vi "FPGA Triggered.vi"(8 "Action":T1, 11 "Input":bool) -> (2 "FPGA Triggered?":bool)   [LabVIEW 2013]
uses:
  <userlib>/Accelerator/Global Variables/Action Items.ctl
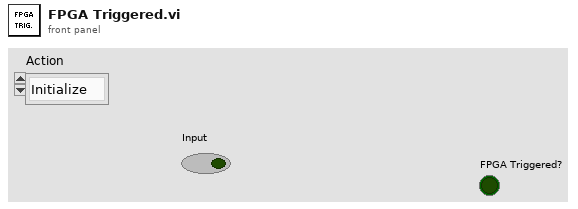
[diagram p1: front panel]
types:
  T1 = typedef "Action Items.ctl" = enum16{"Initialize", "Get", "Set"}
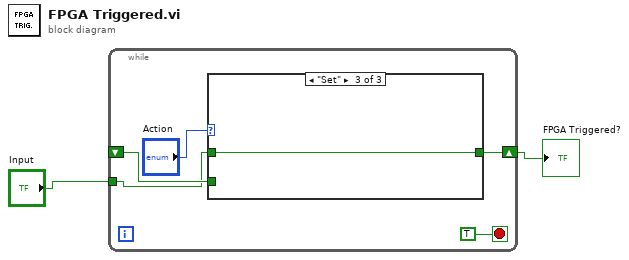
[diagram p0: block diagram]
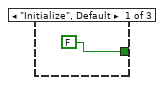
[diagram p2: hidden frame]
diagram:
  n1 = while {
    shift-right: [w5] -> w2
    shift-left: _ -> [w4]
    tunnel: "Input" -> [w3]
    stop <- TRUE stop-if-true
    n2 = case shown="\"Set\"" "Action" {
      tunnel: [FALSE w9 w10] -> w5
      tunnel: w4 -> [_ w9 _]
      tunnel: w3 -> [_ _ w10]
      frame "Initialize", Default {
      }
      frame "Get" {
      }
      frame "Set" {
      }
    }
  }
  "FPGA Triggered?" <- w2
